vi "Chart[Template].ReftoDVR.vi"(10 "Ref":u32 format="%08x") -> (2 "Ref":T1)   [LabVIEW 2020, in "DisplayWaveform.lvlib" / "DisplayWaveforms.lvclass"]
doc: "JKI State Machine Objects (SMO) 1.0.0.5\nJKI - JKI\nCopyright (c) 2016, JKI"
uses:
  DisplayWaveforms.lvclass
  DisplayWaveforms.lvclass/DisplayWaveforms.ctl
  Typedefs/PublicEvents--Cluster.ctl
  Controller/TypeDefs/ChartParamsCluster.ctl
  Typedefs/ProtectedEvents--Cluster.ctl
  Typedefs/Dependencies--Cluster.ctl
  Typedefs/PrivateData--Cluster.ctl
  Typedefs/PrivateData--Ref.ctl
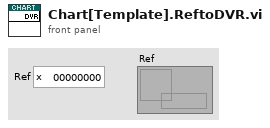
[diagram p1: front panel]
types:
  T1 = typedef "DisplayWaveform.lvlib/DisplayWaveforms.lvclass/PrivateData--Ref.ctl" = refnum<data-value>
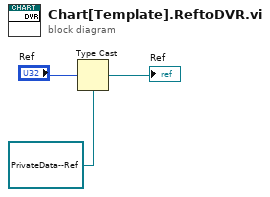
[diagram p0: block diagram]
diagram:
  n1 = Type Cast(type=T1 refnum ("Ref"), x="Ref") -> (*(type *) &x=→"Ref":T1)
